vi "Create Arbitrary Waveform.vi"(6 "Timeout (10000 ms)":u32=10000, 8 "error in (no error)":errorcluster, 9 "Arbitrary Waveform Data":dbl[](array[numeric]), 10 "Arbitrary Waveform Name (\"ARB1\")":string="ARB1", 11 "VISA resource name":refnum<visa-resource-name>) -> (0 "error out":errorcluster, 3 "VISA resource name out":refnum<visa-resource-name>)   [LabVIEW 2012, in "Novatech 409b.lvlib"]
doc: "Creates and saves an arbitrary (user-defined) waveform in non-volatile memory. \n\n<B>Note:</B>\n \n(1) Data is scaled and normalized so that the waveform will be centered around y=0. Models 33120A and 33250A have 12-bit digitizers and will be scaled from -2047 to +2047. Model 33220A has a 14-bit digitizer and will be scaled from -8191 to + 8191.\n\n(2) Call Configure Arbitrary Waveform VI to set the arbitrary waveform as the active function.\n\n(3) Creates an arbitrary waveform in non-volatile memory and because of this, the waveform will remain stored on the instrument until deleted. If any sensitive information is contained in the arbitrary waveform, it is recommended that the waveform be deleted when finished"
uses:
  <instrlib>/Novatech 409b/Novatech 409b.lvlib
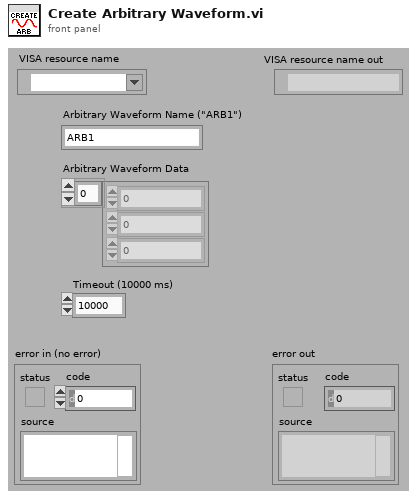
[diagram p1: front panel]
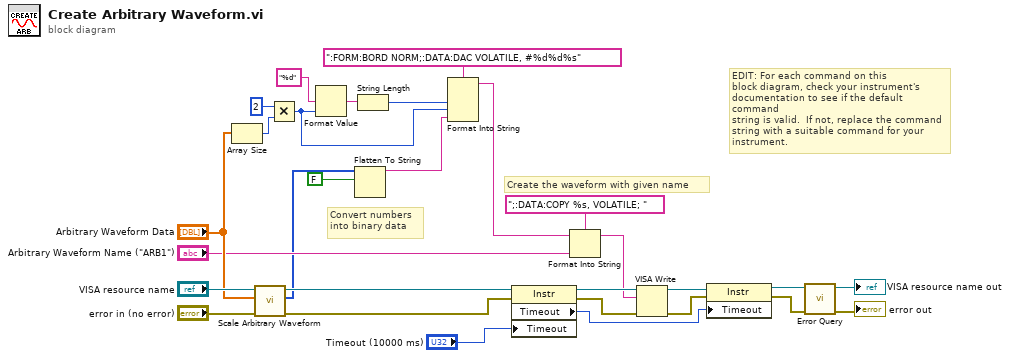
[diagram p0: block diagram]
diagram:
  # "EDIT: For each command on this\nblock diagram, check your instrument's\ndocumentation to see if the default command\nstring is valid.  If not, replace the command\nstring with a suitable command for your\ninstrument."
  # "Convert numbers\ninto binary data"
  # "Create the waveform with given name"
  n1 = Array Size(array="Arbitrary Waveform Data") -> (size(s)=w29:i32)
  n2 = call <instrlib>:"Scale Arbitrary Waveform.vi"("error in (no error)"="error in (no error)", "Arbitrary Waveform Data"="Arbitrary Waveform Data", "VISA resource name"="VISA resource name") -> ("error out"=w22:errorcluster, "Scaled Arbitrary Waveform Data"=w2:i16[], "VISA resource name out"=w23:refnum<visa-resource-name>)  [unwired: 6 in]
  n3 = Multiply(x=2, y=w29) -> (x*y=w13:i32)
  n4 = Format Value(format string="%d", value (0)=w13) -> (output string=w26:string)  [unwired: 1 in]
  n5 = Flatten To String(anything=w2, prepend array or string size? (T)=FALSE) -> (data string=w3:string)  [unwired: 2 in, 2 out]
  n6 = String Length(string=w26) -> (length=w14:i32)
  n7 = Format Into String(format string=":FORM:BORD NORM;:DATA:DAC VOLATILE, #%d%d%s" ("string"), w14, w13, w3) -> (resulting string=w11:string)  [unwired: 2 in, 1 out]
  n8 = property class="Instr"(reference=w23, error in=w22, "Timeout"="Timeout (10000 ms)") -> (reference out=w20:refnum<visa-resource-name>, error out=w21:errorcluster, "Timeout"=w17:u32)
  n9 = Format Into String(format string=";:DATA:COPY %s, VOLATILE; ", initial string=w11, "Arbitrary Waveform Name (\"ARB1\")") -> (resulting string=w9:string)  [unwired: 1 in, 1 out]
  n10 = VISA Write(VISA resource name=w20, write buffer=w9, error in (no error)=w21) -> (VISA resource name out=w19:refnum<visa-resource-name>, error out=w18:errorcluster)  [unwired: 1 out]
  n11 = property class="Instr"(reference=w19, error in=w18, "Timeout"=w17) -> (reference out=w7:refnum<visa-resource-name>, error out=w6:errorcluster)
  n12 = call <instrlib>:"Error Query.vi"("error in (no error)"=w6, "VISA resource name"=w7) -> ("error out"=→"error out":errorcluster, "VISA resource name out"=→"VISA resource name out":refnum<visa-resource-name>)  [unwired: 6 in, 2 out]
